vi "Get Child position from index.vi"(9 "Insertion indent":i32, 10 "Insertion index":i32, 11 "TreeItems (current)":T1[](array[typedef])) -> (1 "Parent Tag Index":i32, 2 "Child Position":i32, 3 "Parent Tag":string)   [LabVIEW 2020, in "BetterDragAndDrop.lvlib" / "BetterTreeHandle.lvclass"]
uses:
  BetterTreeHandle/BetterTreeHandle.lvclass
  TreeItem.ctl
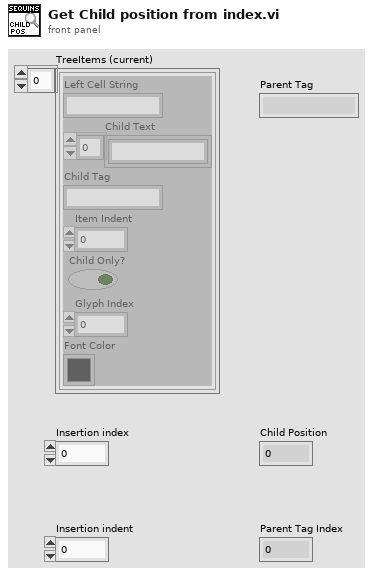
[diagram p1: front panel]
types:
  T1 = typedef "BetterDragAndDrop.lvlib/BetterTreeHandle.lvclass/TreeItem.ctl" = cluster{"Left Cell String":string, "Child Text":string[], "Child Tag":string, "Item Indent":i32, "Child Only?":bool, "Glyph Index":i32, "Font Color":u32}
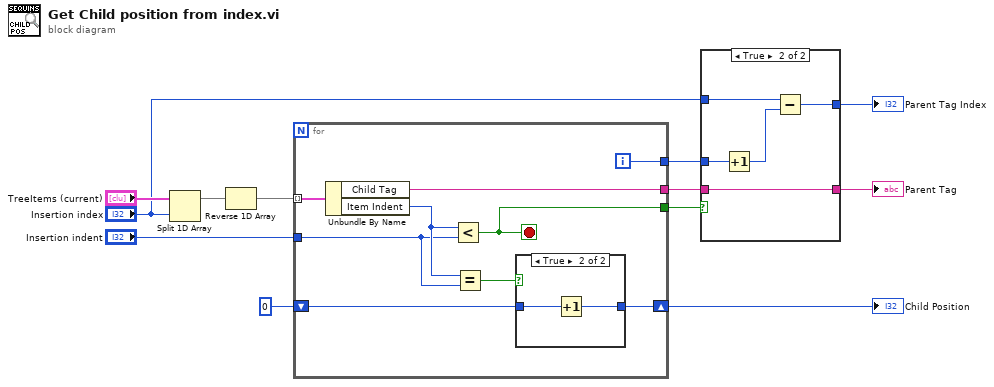
[diagram p0: block diagram]
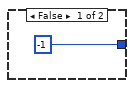
[diagram p2: hidden frame]
diagram:
  n1 = Split 1D Array(array="TreeItems (current)", index="Insertion index") -> (first subarray=w11:T1[])  [unwired: 1 out]
  n2 = Reverse 1D Array(array=w11) -> (reversed array=w10:T1[])
  n3 = for {
    tunnel: w10 -> [w21] mode=indexing
    tunnel: "Insertion indent" -> [w18]
    tunnel: [w20] -> w2
    shift-right: [w15] -> w7
    shift-left: 0 ("Item Indent") -> [w16]
    tunnel: [w14] -> w5
    tunnel: [w13] -> w3
    i -> [w14]
    stop <- w13 stop-if-true
    n4 = Unbundle By Name(w21) -> ("Child Tag"=w20:string, "Item Indent"=w19:i32)
    n5 = Less?(x=w19, y=w18) -> (x < y?=w13:bool)
    n6 = Equal?(x=w19, y=w18) -> (x = y?=w17:bool)
    n7 = case shown="True" w17 {
      tunnel: w16 -> [w22 w24]
      tunnel: [w22 w23] -> w15
      frame False {
      }
      frame True {
        n8 = Increment(x=w24) -> (x+1=w23:i32)
      }
    }
  }
  "Child Position" <- w7
  n9 = case shown="True" w3 {
    tunnel: "Insertion index" -> [_ w30]
    tunnel: w5 -> [_ w27]
    tunnel: [-1 w29] -> w4
    tunnel: w2 -> [_ w28]
    tunnel: [_ w28] -> w1
    frame False {
    }
    frame True {
      n10 = Increment(x=w27) -> (x+1=w26:i32)
      n11 = Subtract(x=w30, y=w26) -> (x-y=w29:i32)
    }
  }
  "Parent Tag" <- w1
  "Parent Tag Index" <- w4
